vi "Write Grid.vi"(8 "error in (no error)":errorcluster, 10 "Grid":u8[][](array[numeric]), 11 "GoL in":refnum<class "GoL.lvclass">) -> (0 "error out":errorcluster, 3 "GoL out":refnum<class "GoL.lvclass">)   [LabVIEW 2026, in "GoL.lvlib" / "GoL.lvclass"]
uses:
  GoL.lvclass
  GoL.lvclass/GoL.ctl
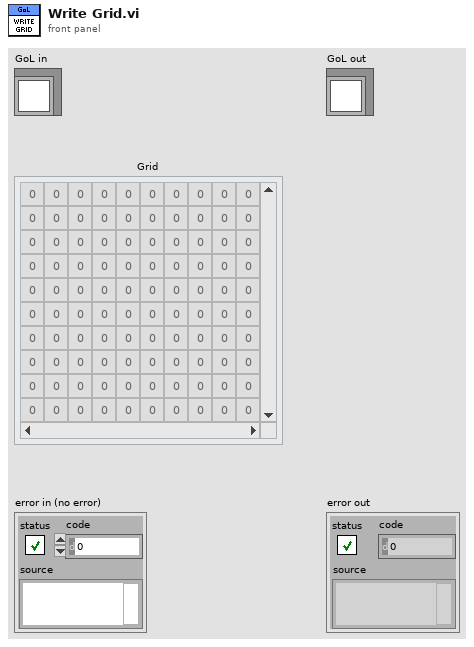
[diagram p1: front panel]
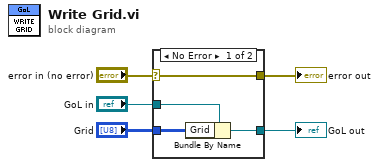
[diagram p0: block diagram]
diagram:
  n1 = case shown="No Error" "error in (no error)" {
    selector: "error in (no error)" -> [w9 w10]
    tunnel: [w9 w10] -> w4
    tunnel: [w7 w11] -> w2
    tunnel: "GoL in" -> [w8 w11]
    tunnel: "Grid" -> [w6 _]
    frame No Error {
      n2 = Bundle By Name(cluster=w8, "Grid"=w6) -> (w7:refnum<class "GoL.lvclass">)
    }
    frame Error {
    }
  }
  "error out" <- w4
  "GoL out" <- w2
